vi "Power Down.vi"(8 "error in":errorcluster, 11 "Neph in":refnum<class "Nephelometer.lvclass">) -> (0 "error out":errorcluster, 3 "Neph out":refnum<class "Nephelometer.lvclass">)   [LabVIEW 2013, in "Nephelometer.lvclass"]
uses:
  Nephelometer.lvclass
  Nephelometer.lvclass/Nephelometer.ctl
  Accessors/Read Session Handle.vi
  Reusable/Session APIs/Serial/Public/Asynchronous Write.vi
  Reusable/Session APIs/Serial/Public/Asynchronous Read.vi
  Reusable/Session APIs/Serial/Serial Session.lvclass
panel:
  out "Read - Asynchronous":string
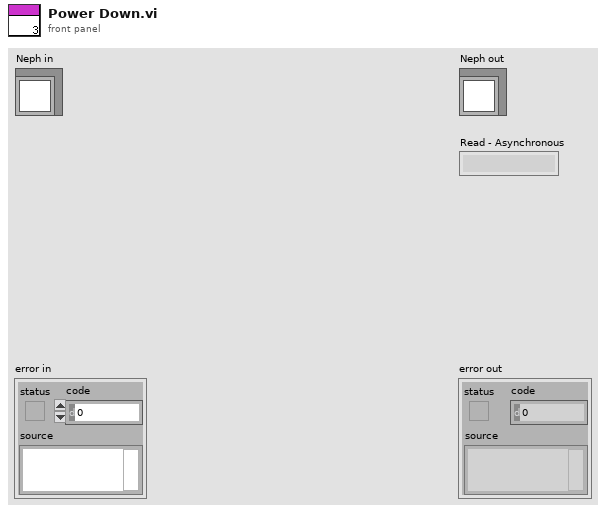
[diagram p1: front panel]
types:
  T1 = typedef "Serial Session.lvclass/Session Handle.ctl" = refnum<data-value>
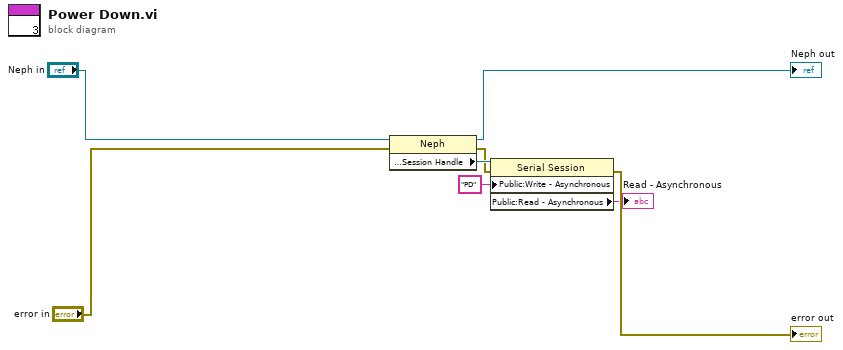
[diagram p0: block diagram]
diagram:
  n1 = property class="Neph"(reference="Neph in", error in="error in") -> (reference out=→"Neph out":refnum<class "Nephelometer.lvclass">, error out=w5:errorcluster, "Accessors:Session Handle"=w7:T1)
  n2 = property class="Serial Session"(reference=w7, error in=w5, "Public:Write - Asynchronous"="PD" ("Write - Asynchronous")) -> (error out=→"error out":errorcluster, "Public:Read - Asynchronous"=→"Read - Asynchronous":string)  [unwired: 1 out]
